vi "数据导出Excel.vi"(8 "error in (no error)":errorcluster caption="错误输入（无错误）", 10 "text data":string[][](array[string]) caption="文本数据", 11 "default name":string="历史数据.xlsx" caption="默认名称") -> (0 "error out":errorcluster caption="错误输出", 3 "布尔":bool)   [LabVIEW 2016, in "数据查询.lvlib"]
uses:
  <vilib>/Utility/sysdir.llb/System Directory Type.ctl
  <vilib>/Utility/file.llb/Write Delimited Spreadsheet (string).vi
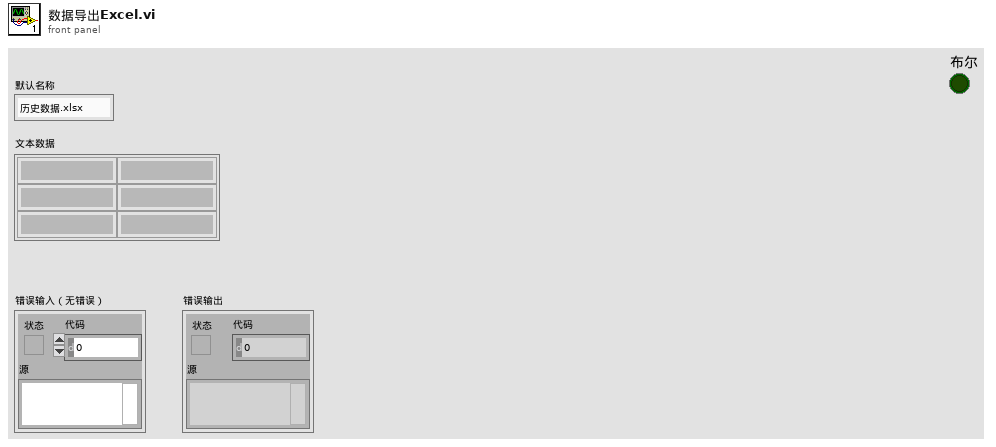
[diagram p1: front panel]
types:
  T1 = typedef "System Directory Type.ctl" = i32
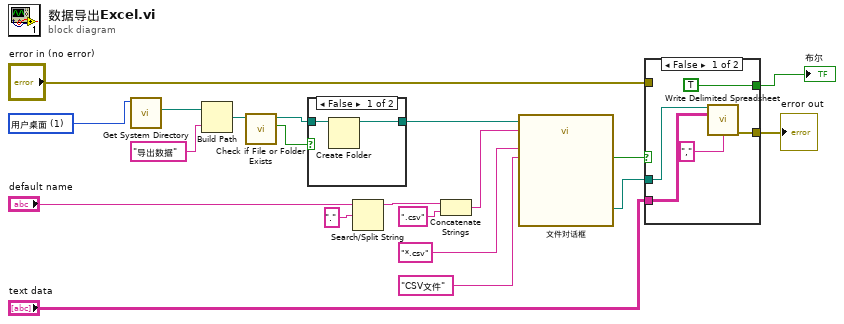
[diagram p0: block diagram]
diagram:
  w7 = T1 1 items=["用户目录"=0, "用户桌面"=1, "用户文档"=2, "用户应用程序数据"=3, "用户设置"=4, "用户临时目录"=5, "公共文档"=6, "公共应用程序数据"=7, "公共设置"=8, "公共缓存"=13, "系统核心库"=9, "系统安装库"=10, "应用程序文件"=11, "启动盘根目录"=12] ("system directory type")
  n1 = call <vilib>:"Get System Directory.vi"("system directory type"=w7) -> ("system directory"=w6:path)  [unwired: 10 in]
  n2 = Build Path(base path=w6, name or relative path="导出数据" ("名称或相对路径")) -> (appended path=w4:path)
  n3 = call <vilib>:"Check if File or Folder Exists.vi"("path"=w4) -> ("file or folder exists?"=w3:bool, "dup path"=w2:path)  [unwired: 8 in, 1 out]
  n4 = case shown="False" w3 {
    tunnel: w2 -> [w22 w23]
    tunnel: [w21 w23] -> w1
    frame False {
      n5 = Create Folder(path (use dialog)=w22) -> (created path=w21:path)  [unwired: 2 in, 2 out]
    }
    frame True {
    }
  }
  n6 = Search/Split String(string="default name", search string/char (-)="." ("搜索字符串/字符(-)")) -> (substring before match=w10:string)  [unwired: 1 in, 2 out]
  n7 = Concatenate Strings(w10, ".csv" ("pattern (all files)")) -> (w8:string)
  n8 = call "文件对话框"("start path"=w1, "default name"=w8, "pattern (all files)"="*.csv", "pattern label"="CSV文件") -> ("selected path"=w17:path, "cancelled"=w18:bool)  [unwired: 8 in, 2 out]
  n9 = case shown="False" w18 {
    tunnel: w17 -> [w27 _]
    tunnel: "error in (no error)" -> [_ w29]
    tunnel: [w24 w29] -> w15
    tunnel: "text data" -> [w26 _]
    tunnel: [TRUE _] -> w13
    frame False {
      n10 = call-poly <vilib>:"Write Delimited Spreadsheet.vi"("file path (dialog if empty)"=w27, "2D data"=w26, "delimiter (\\t)"="," ("delimiter (\\t)")) -> ("error out"=w24:errorcluster)  [unwired: 11 in, 1 out]
    }
    frame True {
    }
  }
  "error out" <- w15
  "布尔" <- w13
